vi "destroy queue pair.vi"(8 "error in":errorcluster, 11 "queue connection":T1) -> (0 "error out":errorcluster)   [LabVIEW 2015, in "Queue connection.lvclass"]
uses:
  Queue connection.lvclass
  queue pair.ctl
  message/communicator message.lvclass
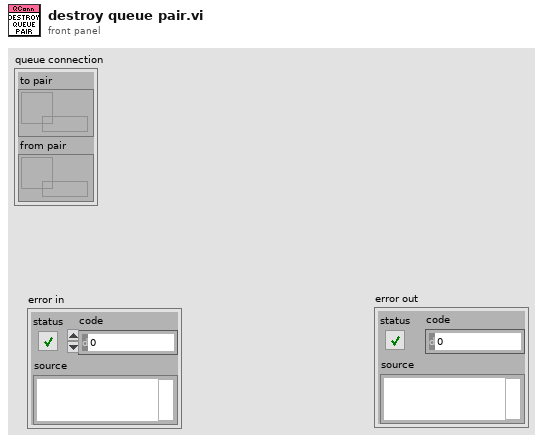
[diagram p1: front panel]
types:
  T1 = typedef "Queue connection.lvclass/queue pair.ctl" = cluster{"to pair":refnum<queue>, "from pair":refnum<queue>}
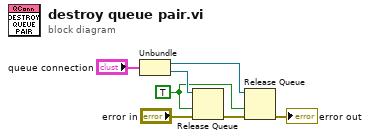
[diagram p0: block diagram]
diagram:
  w1 = TRUE ("force destroy? (F)")
  n1 = Unbundle("queue connection") -> ("to pair"=w5:refnum<queue>, "from pair"=w6:refnum<queue>)
  n2 = Release Queue(queue=w6, force destroy? (F)=w1, error in (no error)="error in") -> (error out=w4:errorcluster)  [unwired: 2 out]
  n3 = Release Queue(queue=w5, force destroy? (F)=w1, error in (no error)=w4) -> (error out=→"error out":errorcluster)  [unwired: 2 out]
